vi "MB Modbus Command to Data Unit.vi"(8 "error in (no error)":errorcluster, 11 "Modbus Command":T1={"Function Code"=1, "Starting Address"=0, "Quantity"=0, "Data"=[], "Discrete"=[]} {"Function Code" items=["Read Discrete Inputs"=2, "Read Coils"=1, "Write Single Coil"=5, "Write Multiple Coils"=15, "Read Input Register"=4, "Read Holding Registers"=3, "Write Single Register"=6, "Write Multiple Registers"=16, "Read/Write Multiple Registers"=23, "Mask Write Register"=22, "Read FIFO Queue"=24, "Read File Record"=20, "Write File Record"=21, "Read Exception Status"=7, "Diagnostic"=8, "Get Com Event Counter"=11, "Get Com Event Log"=12, "Report Slave ID"=17, "Read Device Identification"=43]}) -> (0 "error out":errorcluster, 2 "Modbus Data Unit":T2={"function"=1, "Data"=[]} {"function" items=["Read Discrete Inputs"=2, "Read Coils"=1, "Write Single Coil"=5, "Write Multiple Coils"=15, "Read Input Register"=4, "Read Holding Registers"=3, "Write Single Register"=6, "Write Multiple Registers"=16, "Read/Write Multiple Registers"=23, "Mask Write Register"=22, "Read FIFO Queue"=24, "Read File Record"=20, "Write File Record"=21, "Read Exception Status"=7, "Diagnostic"=8, "Get Com Event Counter"=11, "Get Com Event Log"=12, "Report Slave ID"=17, "Read Device Identification"=43]; "Data" format="%.0x"}, 3 "Quantity":u16)   [LabVIEW 2019, in "NI_modbus_upd.lvlib"]
uses:
  NI_modbus_upd.lvlib
  Ctl/MB Modbus Data Unit.ctl
  Ctl/MB Modbus Command.ctl
  Modbus Data Unit (PDU)/Function.ctl
panel:
  # "VI Name: MB Command to Data Unit\nPurpose: Creates a Modbus Data Unit based on the user's input."
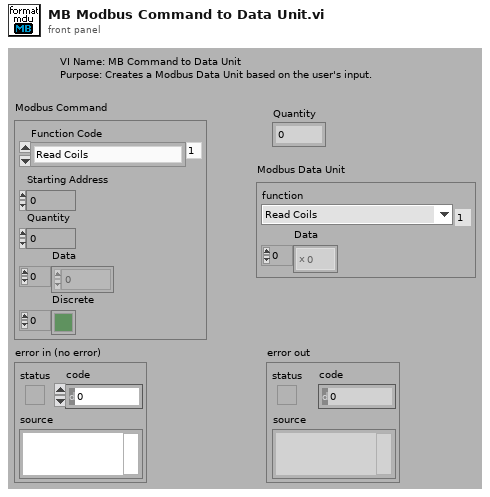
[diagram p1: front panel]
types:
  T1 = typedef "NI_modbus_upd.lvlib/MB Modbus Command.ctl" = cluster{"Function Code":u8, "Starting Address":u16, "Quantity":u16, "Data":u16[], "Discrete":bool[]}
  T2 = typedef "NI_modbus_upd.lvlib/MB Modbus Data Unit.ctl" = cluster{"function":T3, "Data":u8[]}
  T3 = typedef "NI_modbus_upd.lvlib/Function.ctl" = u8
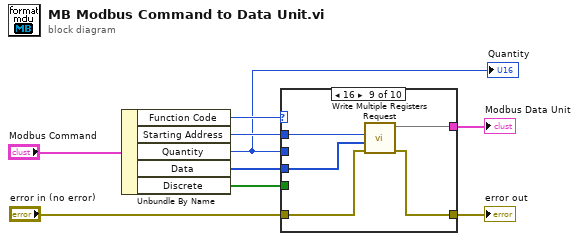
[diagram p0: block diagram]
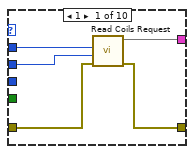
[diagram p2: hidden frame]
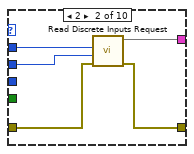
[diagram p3: hidden frame]
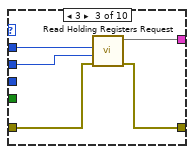
[diagram p4: hidden frame]
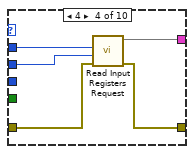
[diagram p5: hidden frame]
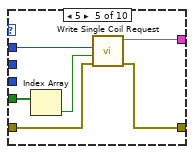
[diagram p6: hidden frame]
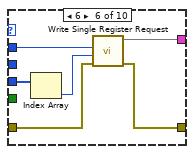
[diagram p7: hidden frame]
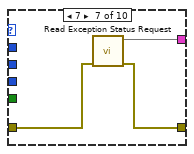
[diagram p8: hidden frame]
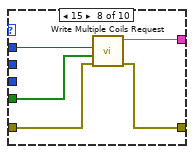
[diagram p9: hidden frame]
diagram:
  n1 = Unbundle By Name("Modbus Command") -> ("Function Code"=w8:u8, "Starting Address"=w7:u16, "Quantity"=w6:u16, "Data"=w5:u16[], "Discrete"=w4:bool[])
  "Quantity" <- w6
  n2 = case shown="16" w8 {
    tunnel: w7 -> [w12 w17 w22 w27 w33 w39 _ w46 w51 _]
    tunnel: w6 -> [w10 w15 w20 w25 _ _ _ _ _ _]
    tunnel: w5 -> [_ _ _ _ _ w37 _ _ w50 _]
    tunnel: w4 -> [_ _ _ _ w31 _ _ w45 _ _]
    tunnel: "error in (no error)" -> [w14 w19 w24 w29 w35 w41 w44 w49 w54 w55]
    tunnel: [w13 w18 w23 w28 w34 w40 w43 w48 w53 w55] -> w2
    tunnel: [w11 w16 w21 w26 w32 w38 w42 w47 w52 _] -> w1
    frame 1 {
      n3 = call "Read Coils Request.vi"("error in (no error)"=w14, "number of coils"=w10, "starting address"=w12) -> ("error out"=w13:errorcluster, 3:w11)  [unwired: 6 in, 1 out]
    }
    frame 2 {
      n4 = call "Read Discrete Inputs Request.vi"("error in (no error)"=w19, "number of inputs"=w15, "starting address"=w17) -> ("error out"=w18:errorcluster, 3:w16)  [unwired: 6 in, 1 out]
    }
    frame 3 {
      n5 = call "Read Holding Registers Request.vi"("error in (no error)"=w24, "number of registers"=w20, "starting address"=w22) -> ("error out"=w23:errorcluster, 3:w21)  [unwired: 6 in, 1 out]
    }
    frame 4 {
      n6 = call "Read Input Registers Request.vi"("error in (no error)"=w29, "number of registers"=w25, "starting address"=w27) -> ("error out"=w28:errorcluster, 3:w26)  [unwired: 6 in, 1 out]
    }
    frame 5 {
      n7 = Index Array(array=w31) -> (element=w30:bool)  [unwired: 1 in]
      n8 = call "Write Single Coil Request.vi"("error in (no error)"=w35, "coil value"=w30, "starting address"=w33) -> ("error out"=w34:errorcluster, 3:w32)  [unwired: 6 in, 1 out]
    }
    frame 6 {
      n9 = Index Array(array=w37) -> (element=w36:u16)  [unwired: 1 in]
      n10 = call "Write Single Register Request.vi"("error in (no error)"=w41, "register value"=w36, "starting address"=w39) -> ("error out"=w40:errorcluster, 3:w38)  [unwired: 6 in, 1 out]
    }
    frame 7 {
      n11 = call "Read Exception Status Request.vi"("error in (no error)"=w44) -> ("error out"=w43:errorcluster, 3:w42)  [unwired: 8 in, 1 out]
    }
    frame 15 {
      n12 = call "Write Multiple Coils Request.vi"("error in (no error)"=w49, "coils to write"=w45, "starting address"=w46) -> ("error out"=w48:errorcluster, 3:w47)  [unwired: 6 in, 1 out]
    }
    frame 16 {
      n13 = call "Write Multiple Registers Request.vi"("error in (no error)"=w54, "registers"=w50, "starting address"=w51) -> ("error out"=w53:errorcluster, 3:w52)  [unwired: 6 in, 1 out]
    }
    frame Default {
    }
  }
  "Modbus Data Unit" <- w1
  "error out" <- w2
